vi "Write Status.vi"(8 "error in (no error)":errorcluster, 10 "Calibration Unit Contents":T1, 11 "Calibration Unit in":refnum<class "Calibration Unit.lvclass">) -> (0 "error out":errorcluster, 3 "Calibration Unit out":refnum<class "Calibration Unit.lvclass">)   [LabVIEW 2018, in "Calibration Unit.lvclass"]
uses:
  Calibration Unit.lvclass
  Calibration Unit.lvclass/Calibration Unit.ctl
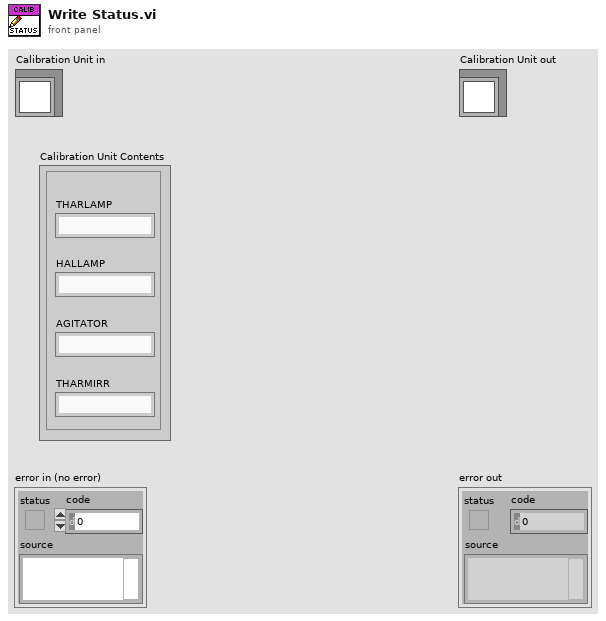
[diagram p1: front panel]
types:
  T1 = cluster{"THARLAMP":string, "HALLAMP":string, "AGITATOR":string, "THARMIRR":string}
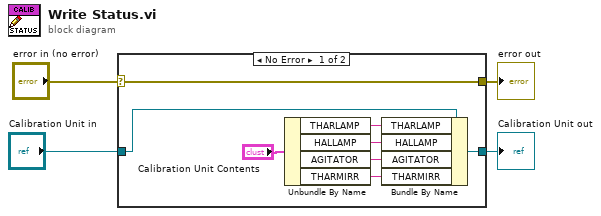
[diagram p0: block diagram]
diagram:
  n1 = case shown="No Error" "error in (no error)" {
    selector: "error in (no error)" -> [w12 w14]
    tunnel: [w12 w14] -> w3
    tunnel: [w10 w13] -> w1
    tunnel: "Calibration Unit in" -> [w11 w13]
    frame No Error {
      n2 = Unbundle By Name("Calibration Unit Contents") -> ("THARLAMP"=w5:string, "HALLAMP"=w6:string, "AGITATOR"=w7:string, "THARMIRR"=w8:string)
      n3 = Bundle By Name(cluster=w11, "THARLAMP"=w5, "HALLAMP"=w6, "AGITATOR"=w7, "THARMIRR"=w8) -> (w10:refnum<class "Calibration Unit.lvclass">)
    }
    frame Error {
    }
  }
  "error out" <- w3
  "Calibration Unit out" <- w1
